vi "Queue Destroy.vi"(8 "error in (no error)":errorcluster, 11 "queue name in":string) -> (0 "error out":errorcluster, 3 "queue name out":string)   [LabVIEW 2020]
uses:
  Control/Queue Data.ctl
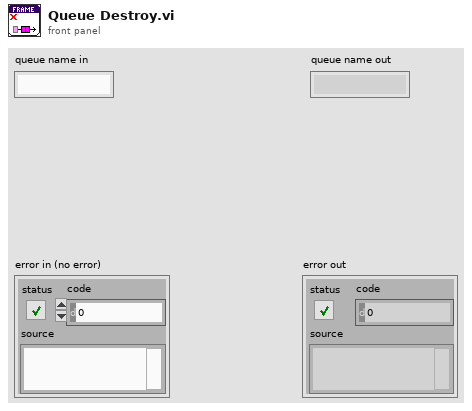
[diagram p1: front panel]
types:
  T1 = typedef "Queue Data.ctl" = cluster{"event":string, "data":variant}
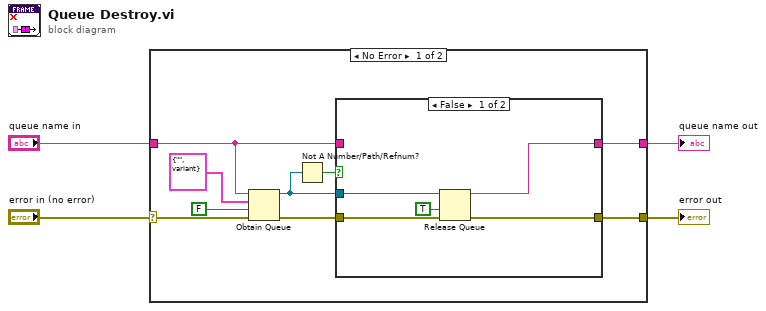
[diagram p0: block diagram]
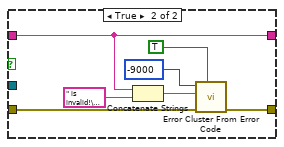
[diagram p2: hidden frame]
diagram:
  n1 = case shown="No Error" "error in (no error)" {
    selector: "error in (no error)" -> [w13 w27]
    tunnel: [w5 w27] -> w3
    tunnel: "queue name in" -> [w7 w26]
    tunnel: [w6 w26] -> w1
    frame No Error {
      n2 = Obtain Queue(name (unnamed)=w7, element data type=T1 {"event"="", "data"=variant}, create if not found? (T)=FALSE, error in (no error)=w13) -> (queue out=w9:refnum<queue>, error out=w10:errorcluster)  [unwired: 1 in, 1 out]
      n3 = Not A Number/Path/Refnum?(number/path/refnum=w9) -> (NaN/Path/Refnum?=w8:bool)
      n4 = case shown="False" w8 {
        tunnel: w10 -> [w18 w21]
        tunnel: w9 -> [w16 _]
        tunnel: w7 -> [_ w20]
        tunnel: [w14 w20] -> w6
        tunnel: [w15 w19] -> w5
        frame False {
          n5 = Release Queue(queue=w16, force destroy? (F)=TRUE, error in (no error)=w18) -> (queue name=w14:string, error out=w15:errorcluster)  [unwired: 1 out]
        }
        frame True {
          n6 = Concatenate Strings(w20, " is invalid!\nEnsure the queue has been created!" ("字符串")) -> (w25:string)
          n7 = call <vilib>:"Error Cluster From Error Code.vi"("show call chain? (False)"=TRUE, "error in (no error)"=w21, "error message (\"\")"=w25, "error code (0)"=-9000) -> ("error out"=w19:errorcluster)  [unwired: 5 in]
        }
      }
    }
    frame Error {
    }
  }
  "error out" <- w3
  "queue name out" <- w1
